vi "SVA 4MV6 T011 CCE3.vi"() -> ()   [LabVIEW 2020]
panel:
  in  "Path":path
  out "2D Picture":picture
  # "Ceballos Conde Emanuel"
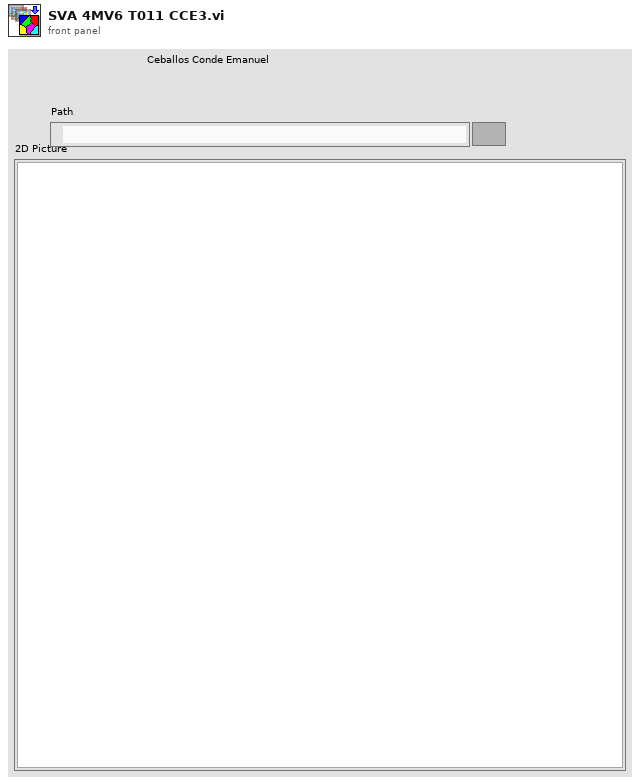
[diagram p1: front panel]
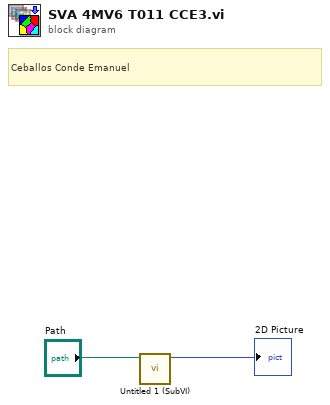
[diagram p0: block diagram]
diagram:
  # "Ceballos Conde Emanuel"
  n1 = call "Untitled 1 (SubVI).vi"("Path"="Path") -> ("new picture"=→"2D Picture":picture)  [unwired: 10 in]
